vi "SVXMPL_Continuous Sine Waveform.vi"(6 "sampling info":cluster{"Fs":dbl, "#s":dbl}={"Fs"=1000.0, "#s"=1000.0} {"#s" format="%.2p"; "Fs" format="%.2p"}, 7 "generation control":T2(ring), 8 "error in":errorcluster, 9 "delay until transition (0 samples)":i32, 10 "current waveform state":T3 {"tf" format="%.2f"; "offset" format="%.2f"; "phase in" format="%.2f"; "amplitude" format="%.2f"; "frequency" format="%.2f"}, 11 "desired waveform state":T1={"frequency"=10.0, "amplitude"=1.0, "offset"=0.0, "phase"=0.0, "tf (ignored)"=0.0} {"tf (ignored)" format="%.2f"; "phase" format="%.2f"; "offset" format="%.2p"; "amplitude" format="%.2p"; "frequency" format="%.2p"}) -> (0 "error out":errorcluster, 1 "index of transition":i32, 2 "next waveform state":T3 {"tf" format="%.2f"; "offset" format="%.2f"; "phase in" format="%.2f"; "amplitude" format="%.2f"; "frequency" format="%.2f"}, 3 "signal out":waveform(dbl))   [LabVIEW 2017]
doc: "Continuous Sine Waveform generates a waveform containing a sine wave. If the frequency or amplitude of the sine wave changes, the VI changes the state of the sine wave at the next available zero crossing."
uses:
  <vilib>/measure/maUtilsandCtls.llb/ma_Updatet0 DBL.vi
  <vilib>/Analysis/NI_AALBase.lvlib
  <vilib>/measure/NI_MABase.lvlib
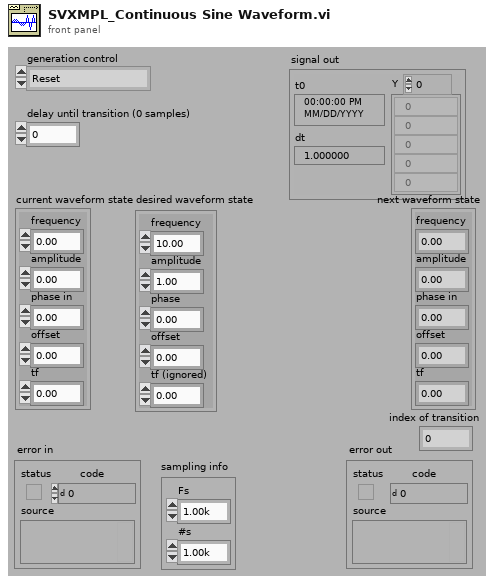
[diagram p1: front panel]
types:
  T1 = cluster{"frequency":dbl, "amplitude":dbl, "offset":dbl, "phase":dbl, "tf (ignored)":dbl}
  T2 = enum16{"Reset", "Continue from previous", "Continue from state", "Zero from previous", "Zero from state"}
  T3 = cluster{"frequency":dbl, "amplitude":dbl, "phase in":dbl, "offset":dbl, "tf":dbl}
  T4 = cluster{"frequency":dbl, "amplitude":dbl, "phase out":dbl, "offset":dbl, "tf new":dbl}
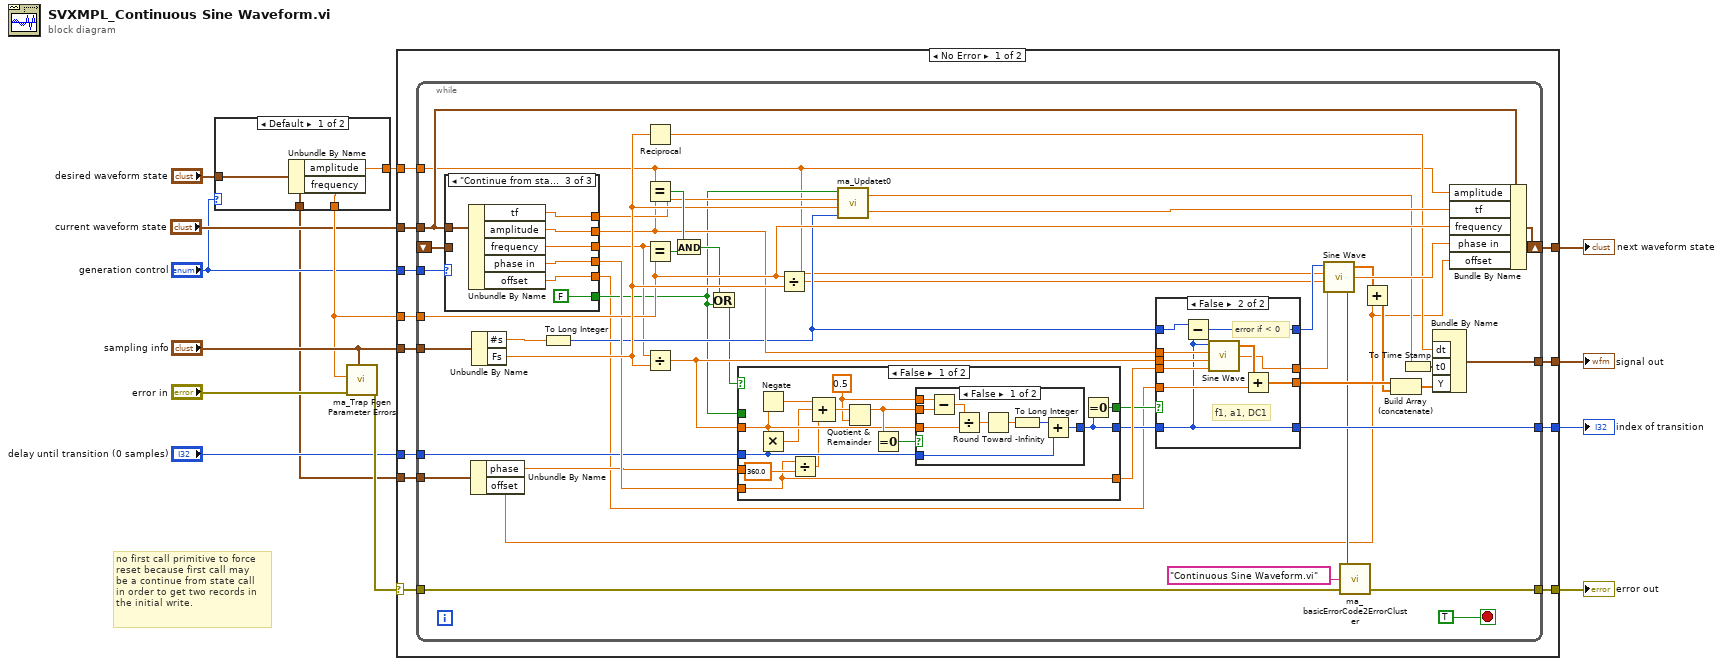
[diagram p0: block diagram]
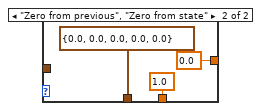
[diagram p2: hidden frame]
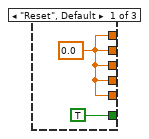
[diagram p3: hidden frame]
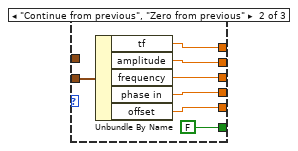
[diagram p4: hidden frame]
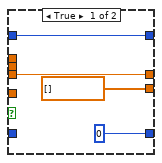
[diagram p5: hidden frame]
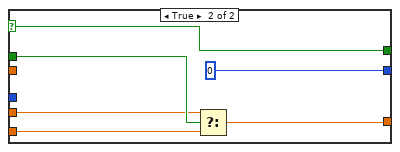
[diagram p7: hidden frame]
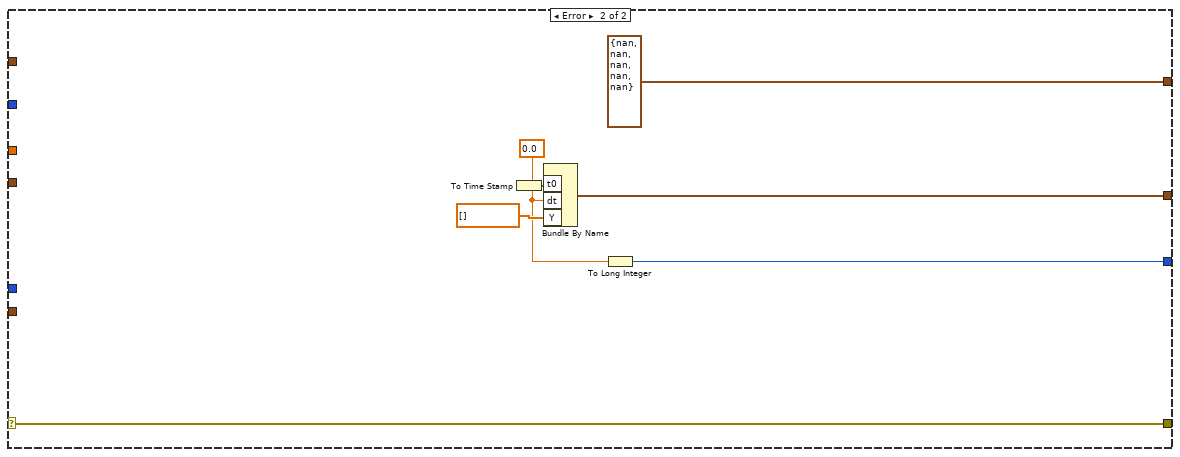
[diagram p8: hidden frame]
diagram:
  # "no first call primitive to force \nreset because first call may \nbe a continue from state call\nin order to get two records in \nthe initial write."
  n1 = case shown="Default" "generation control" {
    tunnel: [w17 0.0 ("amplitude")] -> w7
    tunnel: [w15 1.0 ("frequency")] -> w6
    tunnel: "desired waveform state" -> [w16 _]
    tunnel: [w16 T1 {"frequency"=0.0, "amplitude"=0.0, "offset"=0.0, "phase"=0.0, "tf (ignored)"=0.0} ("desired waveform state")] -> w2
    frame Default {
      n2 = Unbundle By Name(w16) -> ("amplitude"=w17:dbl, "frequency"=w15:dbl)
    }
    frame "Zero from previous", "Zero from state" {
    }
  }
  n3 = call <vilib>:"ma_Trap Fgen Parameter Errors.vi"("Sampling info"="sampling info", "error in (no error)"="error in", "frequency"=w6) -> ("error out"=w11:errorcluster)  [unwired: 8 in]
  n4 = case shown="No Error" w11 {
    selector: w11 -> [w29 w144]
    tunnel: "sampling info" -> [w32 _]
    tunnel: w6 -> [w27 _]
    tunnel: [w31 w144] -> w13
    tunnel: [w30 w145] -> w1
    tunnel: w7 -> [w28 _]
    tunnel: [w26 w141] -> w10
    tunnel: "delay until transition (0 samples)" -> [w25 _]
    tunnel: [w24 T4 {"frequency"=nan, "amplitude"=nan, "phase out"=nan, "offset"=nan, "tf new"=nan}] -> w8
    tunnel: "generation control" -> [w23 _]
    tunnel: w2 -> [w22 _]
    tunnel: "current waveform state" -> [w21 _]
    frame No Error {
      n5 = while {
        tunnel: w21 -> [w41]
        tunnel: w22 -> [w51]
        tunnel: w23 -> [w59]
        shift-left: _ -> [w58]
        shift-right: [w34] -> w24
        tunnel: w25 -> [w48]
        tunnel: [w72] -> w26
        tunnel: w27 -> [w61]
        tunnel: w28 -> [w38]
        tunnel: w29 -> [w75]
        tunnel: [w76] -> w30
        tunnel: [w77] -> w31
        tunnel: w32 -> [w78]
        stop <- TRUE stop-if-true
        n6 = case shown="\"Continue from state\", \"Zero from state\"" w59 {
          tunnel: w58 -> [_ w87 _]
          tunnel: [TRUE FALSE FALSE] -> w43
          tunnel: [w80 w82 w90] -> w57
          tunnel: [w80 w86 w92] -> w56
          tunnel: [w80 w85 w94] -> w46
          tunnel: [w80 w84 w91] -> w55
          tunnel: [w80 w83 w93] -> w37
          tunnel: w41 -> [_ _ w89]
          frame "Reset", Default {
            w80 = 0.0
          }
          frame "Continue from previous", "Zero from previous" {
            n7 = Unbundle By Name(w87) -> ("tf"=w82:dbl, "amplitude"=w86:dbl, "frequency"=w85:dbl, "phase in"=w84:dbl, "offset"=w83:dbl)
          }
          frame "Continue from state", "Zero from state" {
            n8 = Unbundle By Name(w89) -> ("tf"=w90:dbl, "amplitude"=w92:dbl, "frequency"=w94:dbl, "phase in"=w91:dbl, "offset"=w93:dbl)
          }
        }
        n9 = Unbundle By Name(w51) -> ("phase"=w50:dbl, "offset"=w35:dbl)
        n10 = Unbundle By Name(w78) -> ("#s"=w49:dbl, "Fs"=w68:dbl)
        n11 = To Long Integer(number=w49) -> (32bit integer=w52:i32)
        n12 = Reciprocal(x=w68) -> (1/x=w54:dbl)
        n13 = Equal?(x=w38, y=w56) -> (x = y?=w74:bool)
        n14 = Equal?(x=w46, y=w61) -> (x = y?=w73:bool)
        n15 = Divide(x=w46, y=w68) -> (x/y=w67:dbl)
        n16 = And(x=w74, y=w73) -> (x .and. y?=w44:bool)
        n17 = Or(x=w44, y=w43) -> (x .or. y?=w42:bool)
        n18 = case shown="False" w42 {
          selector: w42 -> [_ w138]
          tunnel: [w110 w133] -> w66
          tunnel: w55 -> [w110 w134]
          tunnel: w67 -> [w115 _]
          tunnel: w48 -> [w116 _]
          tunnel: w50 -> [_ w135]
          tunnel: [w121 w138] -> w45
          tunnel: [w119 0] -> w47
          tunnel: w43 -> [_ w136]
          frame False {
            w120 = 0.5 ("y")
            n19 = Negate(x=w115) -> (-x=w114:dbl)
            n20 = Multiply(x=w115, y=w116) -> (x*y=w113:dbl)
            n21 = Divide(x=w110, y=360.0) -> (x/y=w112:dbl)
            n22 = Compound Arithmetic op=ADD(w114, w113, w112) -> (w122:dbl)
            n23 = Quotient & Remainder(x=w122, y=w120) -> (x-y*floor(x/y)=w118:dbl)  [unwired: 1 out]
            n24 = Equal To 0?(x=w118) -> (x = 0?=w117:bool)
            n25 = case shown="False" w117 {
              tunnel: w115 -> [w128 _]
              tunnel: w118 -> [w127 _]
              tunnel: w120 -> [w126 _]
              tunnel: w116 -> [w124 w132]
              tunnel: [w125 w132] -> w119
              frame False {
                n26 = Subtract(x=w126, y=w127) -> (x-y=w129:dbl)
                n27 = Divide(x=w129, y=w128) -> (x/y=w130:dbl)
                n28 = Round Toward -Infinity(1:w130) -> (0:w123:dbl)
                n29 = To Long Integer(number=w123) -> (32bit integer=w131:i32)
                n30 = Add(x=w131, y=w124) -> (x+y=w125:i32)
              }
              frame True {
              }
            }
            n31 = Equal To 0?(x=w119) -> (x = 0?=w121:bool)
          }
          frame True {
            n32 = Select(t=w135, s=w136, f=w134) -> (s? t:f=w133:dbl)
          }
        }
        n33 = Divide(x=w61, y=w68) -> (x/y=w40:dbl)
        n34 = call-poly <vilib>:"ma_Updatet0.vi"("samples"=w52, "sampling rate (S/s)"=w68, "tf previous"=w57, "Reset Generation"=w43) -> ("tf new"=w62:dbl, "t0"=w53:dbl)
        n35 = case shown="False" w45 {
          tunnel: [w97 w100] -> w39
          tunnel: w66 -> [w97 w103]
          tunnel: w52 -> [w96 w104]
          tunnel: w56 -> [_ w109]
          tunnel: [0 w102] -> w72
          tunnel: [dbl[] [] ("Sine Wave") w106] -> w71
          tunnel: [w96 w108] -> w70
          tunnel: w67 -> [_ w107]
          tunnel: w37 -> [_ w105]
          tunnel: w47 -> [_ w102]
          frame True {
          }
          frame False {
            # "error if < 0"
            # "f1, a1, DC1"
            n36 = Subtract(x=w104, y=w102) -> (x-y=w108:i32)
            n37 = call <vilib>:"Sine Wave.vi"("samples"=w102, "amplitude"=w109, "frequency"=w107, "phase in"=w103) -> ("sine wave"=w101:dbl[], "phase out"=w100:dbl)  [unwired: 1 in, 1 out]
            n38 = Add(x=w101, y=w105) -> (x+y=w106:dbl[])
          }
        }
        n39 = call <vilib>:"Sine Wave.vi"("samples"=w70, "amplitude"=w38, "frequency"=w40, "phase in"=w39) -> ("sine wave"=w36:dbl[], "phase out"=w60:dbl, "error"=w69:i32)  [unwired: 1 in]
        n40 = call <vilib>:"ma_basicErrorCode2ErrorCluster.vi"("error in (no error)"=w75, "subVI name"="Continuous Sine Waveform.vi" ("subVI Name"), "Error Code"=w69) -> ("error out"=w77:errorcluster)
        n41 = Add(x=w36, y=w35) -> (x+y=w65:dbl[])
        n42 = Build Array (concatenate)(w71, w65) -> (w64:dbl[])
        n43 = To Time Stamp(1:w53) -> (0:w33:timestamp)
        n44 = Bundle By Name("dt"=w54, "t0"=w33, "Y"=w64) -> (w76:waveform(dbl))  [unwired: 1 in]
        n45 = Bundle By Name(cluster=w41, "amplitude"=w38, "tf"=w62, "frequency"=w61, "phase in"=w60, "offset"=w35) -> (w34:T3)
      }
    }
    frame Error {
      w142 = 0.0 ("t0")
      n46 = To Time Stamp(1:w142) -> (0:w139:timestamp)
      n47 = Bundle By Name("t0"=w139, "dt"=w142, "Y"=dbl[] []) -> (w145:waveform(dbl))  [unwired: 1 in]
      n48 = To Long Integer(number=w142) -> (32bit integer=w141:i32)
    }
  }
  "error out" <- w13
  "signal out" <- w1
  "index of transition" <- w10
  "next waveform state" <- w8
